vi "HW_Stream_raw_data_channel.vi"(8 "error in":errorcluster, 10 "Data flow controls in":T2, 11 "VISA resource name in":refnum<visa-resource-name>) -> (0 "error out":errorcluster, 1 "Output data stream channel":T1, 2 "Data flow controls out":T2, 3 "VISA resource name out":refnum<visa-resource-name>, 4 "Timestamp":timestamp, 5 "Read buffer (for reference only, data is queued)":string)   [LabVIEW 2016]
uses:
  <extravilib>/ChannelInstances/Stream-c(str,stamp)/)Channel.ctl
  <vilib>/Instr/_visa.llb/VISA Flush IO Buffer Mask.ctl
  <extravilib>/ChannelInstances/Stream-c(str,stamp).lvlib
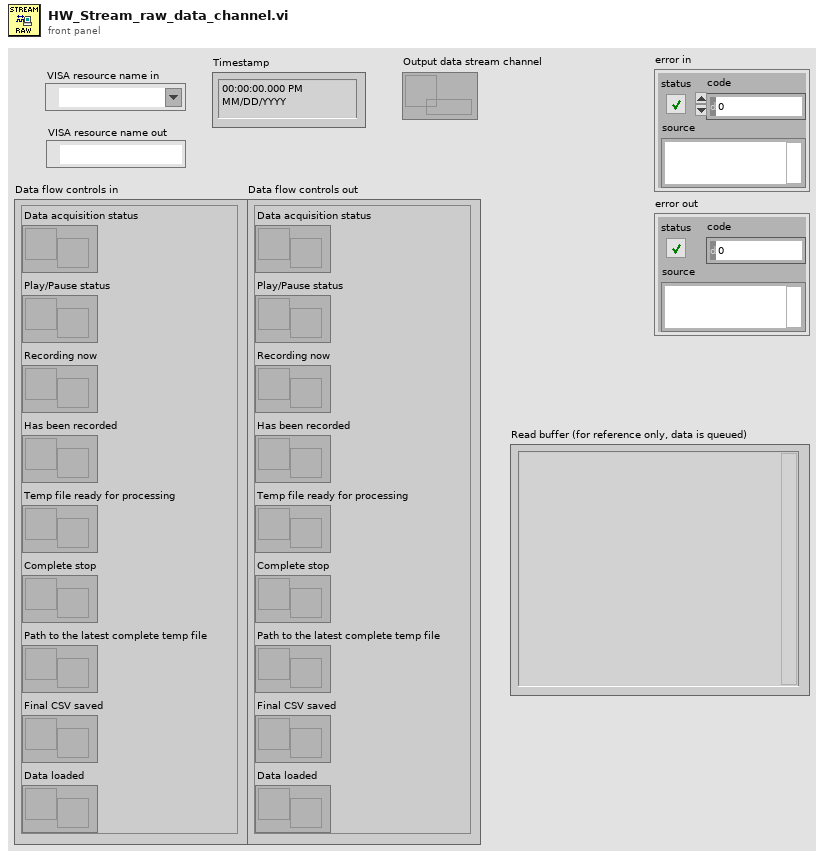
[diagram p1: front panel]
types:
  T1 = typedef "Stream-c(str,stamp).lvlib/)Channel.ctl" = refnum<queue>
  T2 = cluster{"Data acquisition status":refnum<notifier>, "Play/Pause status":refnum<notifier>, "Complete stop":refnum<notifier>, "Temp file ready for processing":refnum<notifier>, "Has been recorded":refnum<notifier>, "Recording now":refnum<notifier>, "Path to the latest complete temp file":refnum<notifier>, "Final CSV saved":refnum<notifier>, "Data loaded":refnum<notifier>}
  T3 = typedef "VISA Flush IO Buffer Mask.ctl" = u16
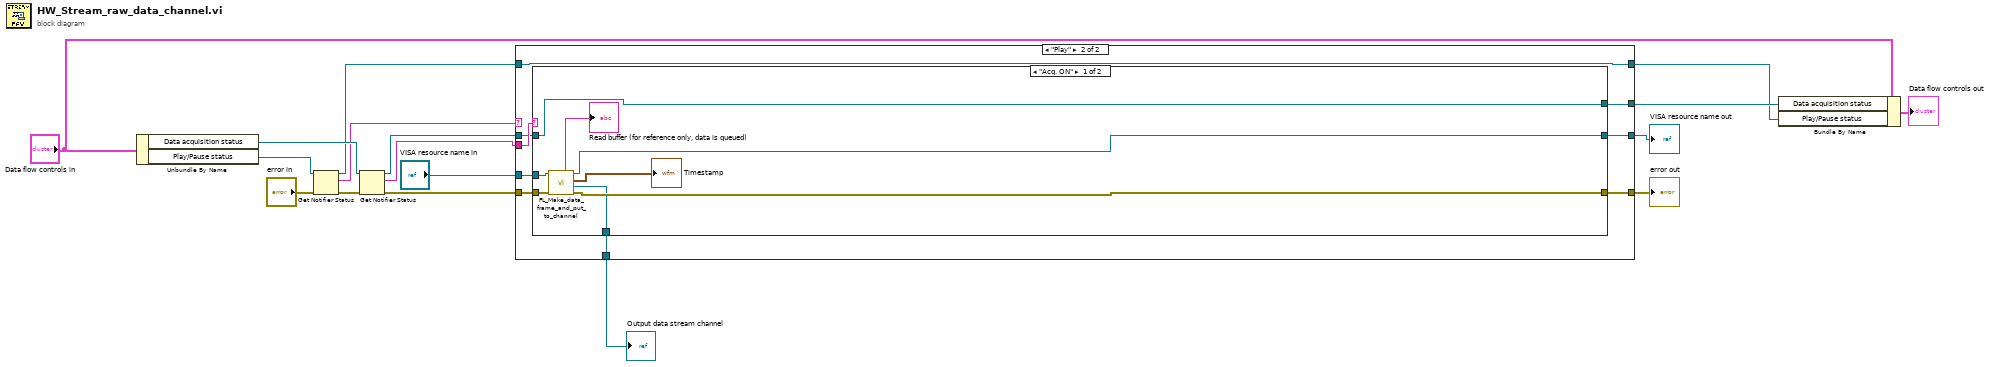
[diagram p0: block diagram]
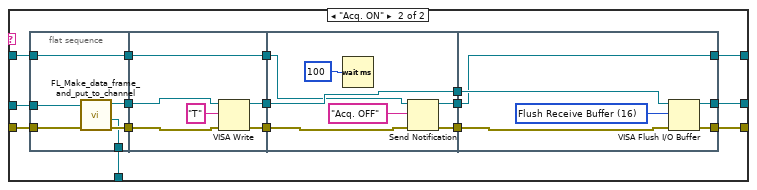
[diagram p3: hidden frame]
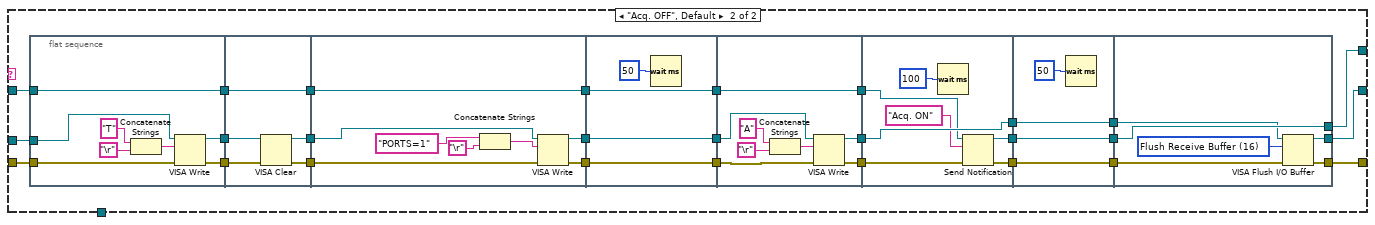
[diagram p4: hidden frame]
diagram:
  n1 = Unbundle By Name("Data flow controls in") -> ("Data acquisition status"=w15:refnum<notifier>, "Play/Pause status"=w14:refnum<notifier>)
  n2 = Get Notifier Status(notifier=w14, error in (no error)="error in") -> (notifier out=w9:refnum<notifier>, current notification=w13:string, error out=w10:errorcluster)  [unwired: 2 out]
  n3 = Get Notifier Status(notifier=w15, error in (no error)=w10) -> (notifier out=w8:refnum<notifier>, current notification=w12:string, error out=w3:errorcluster)  [unwired: 2 out]
  n4 = case shown="\"Play\"" w13 {
    tunnel: [w21 w74] -> w16
    tunnel: "VISA resource name in" -> [w26 w79]
    tunnel: w12 -> [w25 w77]
    tunnel: w9 -> [w23 w75]
    tunnel: w8 -> [w24 w76]
    tunnel: [w20 w73] -> w6
    tunnel: [w23 w75] -> w5
    tunnel: w3 -> [w22 w78]
    tunnel: [w19 w72] -> w2
    tunnel: [w18 w71] -> w1
    frame "Pause", Default {
      n5 = case shown="\"Acq. OFF\", Default" w25 {
        tunnel: w26 -> [w29 w43]
        tunnel: [w29 w42] -> w21
        tunnel: w24 -> [w28 w36]
        tunnel: [w28 w35] -> w20
        tunnel: w22 -> [w27 w39]
        tunnel: [w27 w38] -> w19
        tunnel: [_ w30] -> w18
        frame "Acq. OFF", Default {
        }
        frame "Acq. ON" {
          n6 = flat-sequence {
            tunnel: w36 -> [w51]
            tunnel: w39 -> [w50]
            tunnel: w43 -> [w48]
            tunnel: [w47] -> w33
            tunnel: [w49] -> w32
            tunnel: [w51] -> w31
            tunnel: [w46] -> w30
            tunnel: [w56] -> w45
            tunnel: [w55] -> w44
            tunnel: [w53] -> w37
            tunnel: w33 -> [w57]
            tunnel: w32 -> [w54]
            tunnel: w31 -> [w53]
            tunnel: w45 -> [w63]
            tunnel: w44 -> [w62]
            tunnel: [w63] -> w41
            tunnel: [w61] -> w40
            tunnel: w37 -> [w59]
            tunnel: [w58] -> w34
            tunnel: [w68] -> w42
            tunnel: w41 -> [w69]
            tunnel: w40 -> [w70]
            tunnel: [w66] -> w38
            tunnel: [w65] -> w35
            tunnel: w34 -> [w65]
            frame #0 {
              n7 = call "FL_Make_data_frame_and_put_to_channel.vi"("error in"=w50, "VISA resource name in"=w48) -> ("error out"=w49:errorcluster, "Output data stream channel"=w46:T1, "VISA resource name out"=w47:refnum<visa-resource-name>)  [unwired: 5 in, 2 out]
            }
            frame #1 {
              n8 = VISA Write(VISA resource name=w57, write buffer="T", error in (no error)=w54) -> (VISA resource name out=w56:refnum<visa-resource-name>, error out=w55:errorcluster)  [unwired: 1 out]
            }
            frame #2 {
              n9 = Wait (ms)(milliseconds to wait=u32 100) -> ()  [unwired: 1 out]
              n10 = Send Notification(notification="Acq. OFF", notifier=w59, error in (no error)=w62) -> (notifier out=w58:refnum<notifier>, error out=w61:errorcluster)
            }
            frame #3 {
              w67 = T3 16 items=["Flush Receive Buffer"=16, "Write Transmit Buffer to Device"=32, "Flush Receive Buffer (No I/O)"=64, "Flush Transmit Buffer"=128] ("Mask")
              n11 = VISA Flush I/O Buffer(VISA resource name=w69, mask (16)=w67, error in (no error)=w70) -> (VISA resource name out=w68:refnum<visa-resource-name>, error out=w66:errorcluster)
            }
          }
        }
      }
    }
    frame "Play" {
      n12 = case shown="\"Acq. ON\"" w77 {
        tunnel: w79 -> [w86 w112]
        tunnel: [w81 w111] -> w74
        tunnel: [w82 w110] -> w72
        tunnel: w78 -> [w84 w103]
        tunnel: w76 -> [w87 w98]
        tunnel: [w87 w97] -> w73
        tunnel: [w80 _] -> w71
        frame "Acq. ON" {
          n13 = call "FL_Make_data_frame_and_put_to_channel.vi"("error in"=w84, "VISA resource name in"=w86) -> ("error out"=w82:errorcluster, "Output data stream channel"=w80:T1, "Timestamp"=→"Timestamp":timestamp, "VISA resource name out"=w81:refnum<visa-resource-name>, "Read buffer (for reference only, data is queued)"=→"Read buffer (for reference only, data is queued)":string)  [unwired: 5 in]
        }
        frame "Acq. OFF", Default {
          n14 = flat-sequence {
            tunnel: w112 -> [w121]
            tunnel: [w122] -> w109
            tunnel: [w120] -> w108
            tunnel: w103 -> [w116]
            tunnel: [w115] -> w99
            tunnel: w98 -> [w115]
            tunnel: [w127] -> w105
            tunnel: [w126] -> w104
            tunnel: w108 -> [w125]
            tunnel: w109 -> [w124]
            tunnel: [w123] -> w100
            tunnel: w99 -> [w123]
            tunnel: w105 -> [w133]
            tunnel: [w132] -> w107
            tunnel: w104 -> [w131]
            tunnel: [w130] -> w106
            tunnel: [w128] -> w101
            tunnel: w100 -> [w128]
            tunnel: [w138] -> w90
            tunnel: [w137] -> w89
            tunnel: [w139] -> w88
            tunnel: w101 -> [w139]
            tunnel: w107 -> [w138]
            tunnel: w106 -> [w137]
            tunnel: [w142] -> w114
            tunnel: [w141] -> w113
            tunnel: w90 -> [w144]
            tunnel: w89 -> [w143]
            tunnel: [w140] -> w102
            tunnel: w88 -> [w140]
            tunnel: w114 -> [w152]
            tunnel: w113 -> [w153]
            tunnel: w102 -> [w150]
            tunnel: [w151] -> w96
            tunnel: [w153] -> w95
            tunnel: [w149] -> w94
            tunnel: w96 -> [w158]
            tunnel: [w158] -> w93
            tunnel: w95 -> [w157]
            tunnel: [w157] -> w92
            tunnel: w94 -> [w156]
            tunnel: [w156] -> w91
            tunnel: [w160] -> w97
            tunnel: [w164] -> w111
            tunnel: [w163] -> w110
            tunnel: w91 -> [w160]
            tunnel: w92 -> [w159]
            tunnel: w93 -> [w161]
            frame #0 {
              n15 = Concatenate Strings("T" ("write buffer"), "\r") -> (w117:string)
              n16 = VISA Write(VISA resource name=w121, write buffer=w117, error in (no error)=w116) -> (VISA resource name out=w122:refnum<visa-resource-name>, error out=w120:errorcluster)  [unwired: 1 out]
            }
            frame #1 {
              n17 = VISA Clear(VISA resource name=w124, error in (no error)=w125) -> (VISA resource name out=w127:refnum<visa-resource-name>, error out=w126:errorcluster)
            }
            frame #2 {
              n18 = Concatenate Strings("PORTS=1" ("write buffer"), "\r") -> (w134:string)
              n19 = VISA Write(VISA resource name=w133, write buffer=w134, error in (no error)=w131) -> (VISA resource name out=w132:refnum<visa-resource-name>, error out=w130:errorcluster)  [unwired: 1 out]
            }
            frame #3 {
              n20 = Wait (ms)(milliseconds to wait=u32 50) -> ()  [unwired: 1 out]
            }
            frame #4 {
              n21 = Concatenate Strings("A" ("write buffer"), "\r") -> (w145:string)
              n22 = VISA Write(VISA resource name=w144, write buffer=w145, error in (no error)=w143) -> (VISA resource name out=w141:refnum<visa-resource-name>, error out=w142:errorcluster)  [unwired: 1 out]
            }
            frame #5 {
              n23 = Wait (ms)(milliseconds to wait=u32 100) -> ()  [unwired: 1 out]
              n24 = Send Notification(notification="Acq. ON", notifier=w150, error in (no error)=w152) -> (notifier out=w149:refnum<notifier>, error out=w151:errorcluster)
            }
            frame #6 {
              n25 = Wait (ms)(milliseconds to wait=u32 50) -> ()  [unwired: 1 out]
            }
            frame #7 {
              w162 = T3 16 items=["Flush Receive Buffer"=16, "Write Transmit Buffer to Device"=32, "Flush Receive Buffer (No I/O)"=64, "Flush Transmit Buffer"=128] ("Mask")
              n26 = VISA Flush I/O Buffer(VISA resource name=w159, mask (16)=w162, error in (no error)=w161) -> (VISA resource name out=w164:refnum<visa-resource-name>, error out=w163:errorcluster)
            }
          }
        }
      }
    }
  }
  "VISA resource name out" <- w16
  "error out" <- w2
  "Output data stream channel" <- w1
  n27 = Bundle By Name(cluster="Data flow controls in", "Data acquisition status"=w6, "Play/Pause status"=w5) -> (→"Data flow controls out":T2)
